vi "自动计算参数.vi"(8 "功率控制表":refnum<vi>, 9 "标定参数表":refnum<vi>, 11 "应用程序输入":refnum<vi>) -> ()   [LabVIEW 2015]
uses:
  <vilib>/addons/_office/excel.llb/Excel Easy Table (str).vi
  <vilib>/addons/_office/excel.llb/Excel Get Data ([str]).vi
  <vilib>/Utility/NIReport.llb/NI_report.lvclass
  <vilib>/addons/_office/NI_ReportGenerationToolkit.lvlib
  <vilib>/Utility/NIReport.llb/Excel/NI_Excel.lvclass
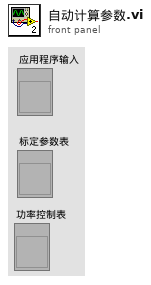
[diagram p1: front panel]
types:
  T1 = enum16{"Standard Report", "HTML", "Word", "Excel"}
  T2 = enum16{"maximized", "minimized", "normal", "no change"}
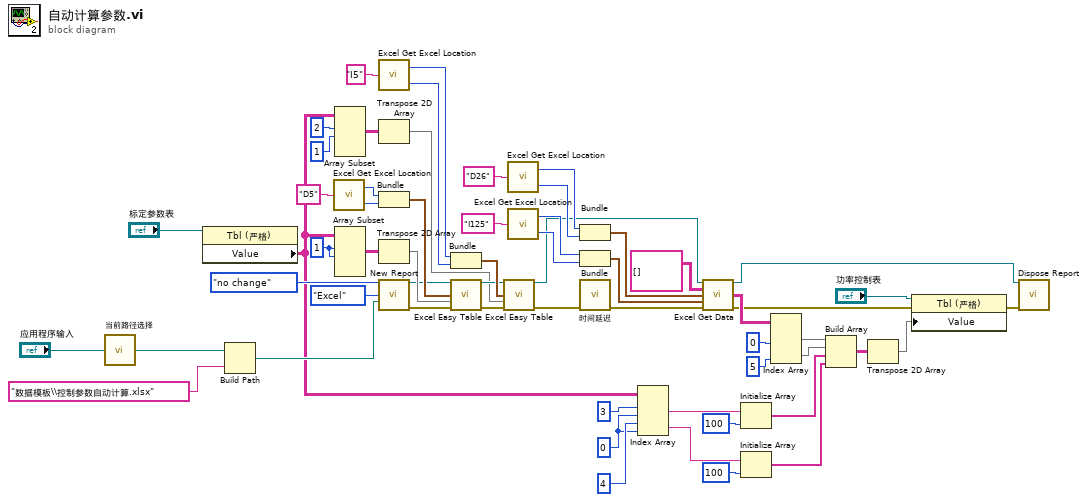
[diagram p0: block diagram]
diagram:
  w16 = 0 ("索引 (行)")
  w33 = 1 ("索引 (行)")
  n1 = call "当前路径选择.vi"("本应用程序"="应用程序输入") -> ("当前路径"=w29:path)
  n2 = property class="Tbl (严格)"(reference="标定参数表") -> ("Value"=w19:string[][])  [unwired: 1 in, 2 out]
  n3 = Build Path(base path=w29, name or relative path="数据模板\\控制参数自动计算.xlsx" ("名称或相对路径")) -> (appended path=w30:path)
  n4 = call <vilib>:"Excel Get Excel Location.vi"("cell's name"="D5") -> ("row"=w37:i32, "column"=w38:i32)
  n5 = Array Subset(array=w19, index (row)=2 ("索引 (行)"), length (row)=1 ("索引 (行)")) -> (w49:string[][])  [unwired: 2 in]
  n6 = Array Subset(array=w19, index (row)=w33, length (row)=w33) -> (w34:string[][])  [unwired: 2 in]
  n7 = call <vilib>:"Excel Get Excel Location.vi"("cell's name"="I5") -> ("row"=w44:i32, "column"=w43:i32)
  n8 = Transpose 2D Array(2D array=w49) -> (transposed array=w4:string[][])
  n9 = Bundle("row"=w37, "column"=w38) -> (w39:cluster{"row":i32, "column":i32})  [unwired: 1 in]
  n10 = Transpose 2D Array(2D array=w34) -> (transposed array=w35:string[][])
  n11 = call <vilib>:"New Report.vi"("window state (normal)"=T2."no change", "report type"=T1."Excel", "template (empty)"=w30) -> ("report out"=w31:refnum<class "NI_report.lvclass">, "error out"=w32:errorcluster)  [unwired: 11 in]
  n12 = Bundle("row"=w44, "column"=w43) -> (w46:cluster{"row":i32, "column":i32})  [unwired: 1 in]
  n13 = call-poly <vilib>:"Excel Easy Table.vi"("report in"=w31, "start (0, 0)"=w39, "text data"=w35, "error in (no error)"=w32) -> ("report out"=w42:refnum<class "NI_report.lvclass">, "error out"=w41:errorcluster)  [unwired: 7 in, 3 out]
  n14 = call-poly <vilib>:"Excel Easy Table.vi"("report in"=w42, "start (0, 0)"=w46, "text data"=w4, "error in (no error)"=w41) -> ("report out"=w50:refnum<class "NI_report.lvclass">, "error out"=w2:errorcluster)  [unwired: 7 in, 3 out]
  n15 = call <vilib>:"Excel Get Excel Location.vi"("cell's name"="D26") -> ("row"=w53:i32, "column"=w52:i32)
  n16 = call <vilib>:"Excel Get Excel Location.vi"("cell's name"="I125") -> ("row"=w55:i32, "column"=w56:i32)
  n17 = Bundle("row"=w53, "column"=w52) -> (w54:cluster{"row":i32, "column":i32})  [unwired: 1 in]
  n18 = Bundle("row"=w55, "column"=w56) -> (w58:cluster{"row":i32, "column":i32})  [unwired: 1 in]
  n19 = call "时间延迟"("error in (no error)"=w2) -> ("error out"=w1:errorcluster)  [unwired: 10 in]
  n20 = Index Array(array=w19, index (row) #1=3 ("索引 (行)"), index (col) #1=w16, index (row) #2=4 ("索引 (行)"), index (col) #2=w16) -> (element #1=w15:string, element #2=w12:string)
  n21 = call-poly <vilib>:"Excel Get Data.vi"("report in"=w50, "data type"=string[][] [], "start (-1, -1)"=w54, "end (-1, -1)"=w58, "error in (no error)"=w1) -> ("report out"=w6:refnum<class "NI_report.lvclass">, "data"=w24:string[][], "error out"=w8:errorcluster)  [unwired: 8 in]
  n22 = Initialize Array(w15, 100 ("维数大小")) -> (w11:string[])
  n23 = Initialize Array(w12, 100 ("维数大小")) -> (w10:string[])
  n24 = Index Array(array=w24, index (col) #1=0 ("禁用的索引 (列)"), index (col) #2=5 ("禁用的索引 (列)")) -> (element #1=w21:string[], element #2=w20:string[])  [unwired: 2 in]
  n25 = Build Array(w21, w20, w11, w10) -> (w9:string[][])
  n26 = Transpose 2D Array(2D array=w9) -> (transposed array=w3:string[][])
  n27 = property class="Tbl (严格)"(reference="功率控制表", error in=w8, "Value"=w3) -> (error out=w7:errorcluster)  [unwired: 1 out]
  n28 = call-dynamic "Dispose Report.vi"("report in"=w6, "error in (no error)"=w7) -> ()  [unwired: 13 in, 1 out]
